vi "U8ToU16.vi"(4 "Index":u32, 7 "Input U8 Array":u8[](array[numeric])) -> (0 "Index+2":u32, 1 "Output U16":u16, 3 "Output U8 Array":u8[](array[numeric]))   [LabVIEW 2017]
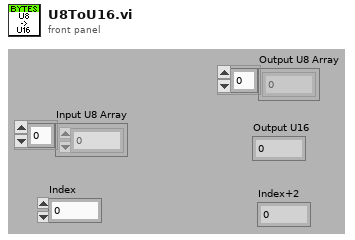
[diagram p1: front panel]
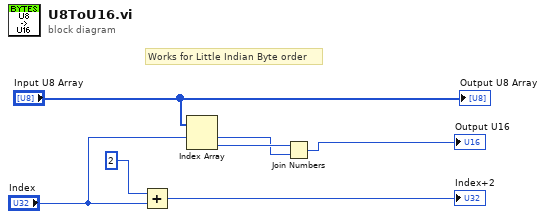
[diagram p0: block diagram]
diagram:
  # "Works for Little Indian Byte order"
  n1 = Add(x=2 ("count (1)"), y="Index") -> (x+y=→"Index+2":u32)
  n2 = Index Array(array="Input U8 Array", index #1="Index") -> (element #1=w6:u8, element #2=w7:u8)  [unwired: 1 in]
  n3 = Join Numbers(hi=w7, lo=w6) -> ((hi.lo)=→"Output U16":u16)
  "Output U8 Array" <- "Input U8 Array"
